vi "harp_read_reg.vi"(0 "port":refnum<visa-resource-name>, 5 "error in (no error)":errorcluster, 6 "port":u8, 8 "reg. address":u8, 9 "type":u8(ring)=1 items=["U8"=1, "U16"=2, "U32 "=4, "U64"=8, "I8"=129, "I16"=130, "I32"=132, "I64"=136, "FLOAT"=68, "BOOL"=17]) -> (10 "HarpDataFrame":T1={"Timestamp(us)"=0.0, "Command"=16, "Error"=FALSE, "Register Address"=16, "Port"=16, "Number of Elements"=16, "Type"=16, "I8"=0, "U8"=0, "U16"=0, "I16"=0, "U32"=0, "I32"=0, "U64"=0, "I64"=0, "Float"=0.0, "U8[]"=[], "I8[]"=[], "U16[]"=[], "I16[]"=[], "U32[]"=[], "I32[]"=[], "U64[]"=[], "I64[]"=[], "Float[]"=[]} {"Timestamp(us)" format="%.6f"}, 11 "timestamp":dbl format="%.6f", 12 "8 bits":u8 format="%x", 13 "bool":bool, 14 "port out":refnum<visa-resource-name>, 15 "16 bits":u16, 16 "32 bits":u32, 17 "64 bits":u64, 18 "float":sgl, 19 "error out":errorcluster)   [LabVIEW 2010]
uses:
  <vilib>/Instr/_visa.llb/VISA Flush IO Buffer Mask.ctl
panel:
  out "Float":sgl
  out "U64":u64
  out "U32":u32
  out "U16":u16
  out "U8":u8
  out "I64":i64
  out "I32":i32
  out "I16":i16
  out "I8":i8
  out "U8[]":u8[](array[numeric])
  out "I8[]":i8[](array[numeric])
  out "U16[]":u16[](array[numeric])
  out "I16[]":i16[](array[numeric])
  out "U32[]":u32[](array[numeric])
  out "I32[]":i32[](array[numeric])
  out "U64[]":u64[](array[numeric])
  out "I64[]":i64[](array[numeric])
  out "Float[]":sgl[](array[numeric])
  in  "Round value":bool
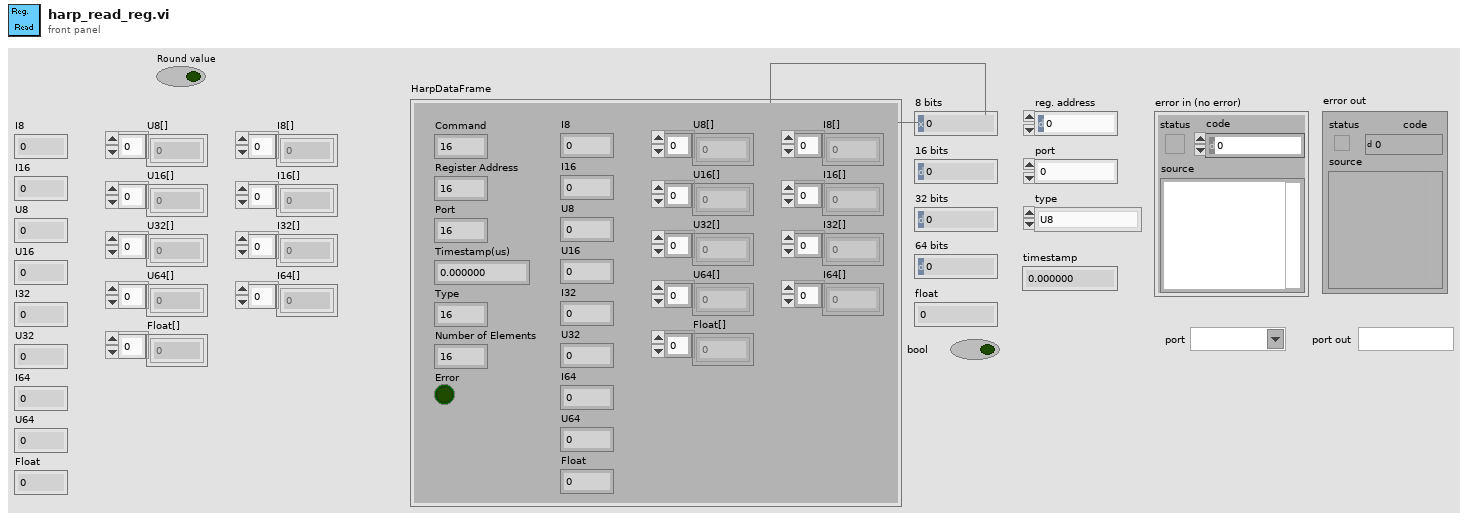
[diagram p1: front panel]
types:
  T1 = cluster{"Timestamp(us)":dbl, "Command":u8, "Error":bool, "Register Address":u8, "Port":u8, "Number of Elements":u8, "Type":u8, "I8":i8, "U8":u8, "U16":u16, "I16":i16, "U32":u32, "I32":i32, "U64":u64, "I64":i64, "Float":sgl, "U8[]":u8[], "I8[]":i8[], "U16[]":u16[], "I16[]":i16[], "U32[]":u32[], "I32[]":i32[], "U64[]":u64[], "I64[]":i64[], "Float[]":sgl[]}
  T2 = typedef "VISA Flush IO Buffer Mask.ctl" = u16
  T3 = enum16{"big-endian, network order", "native, host order", "little-endian"}
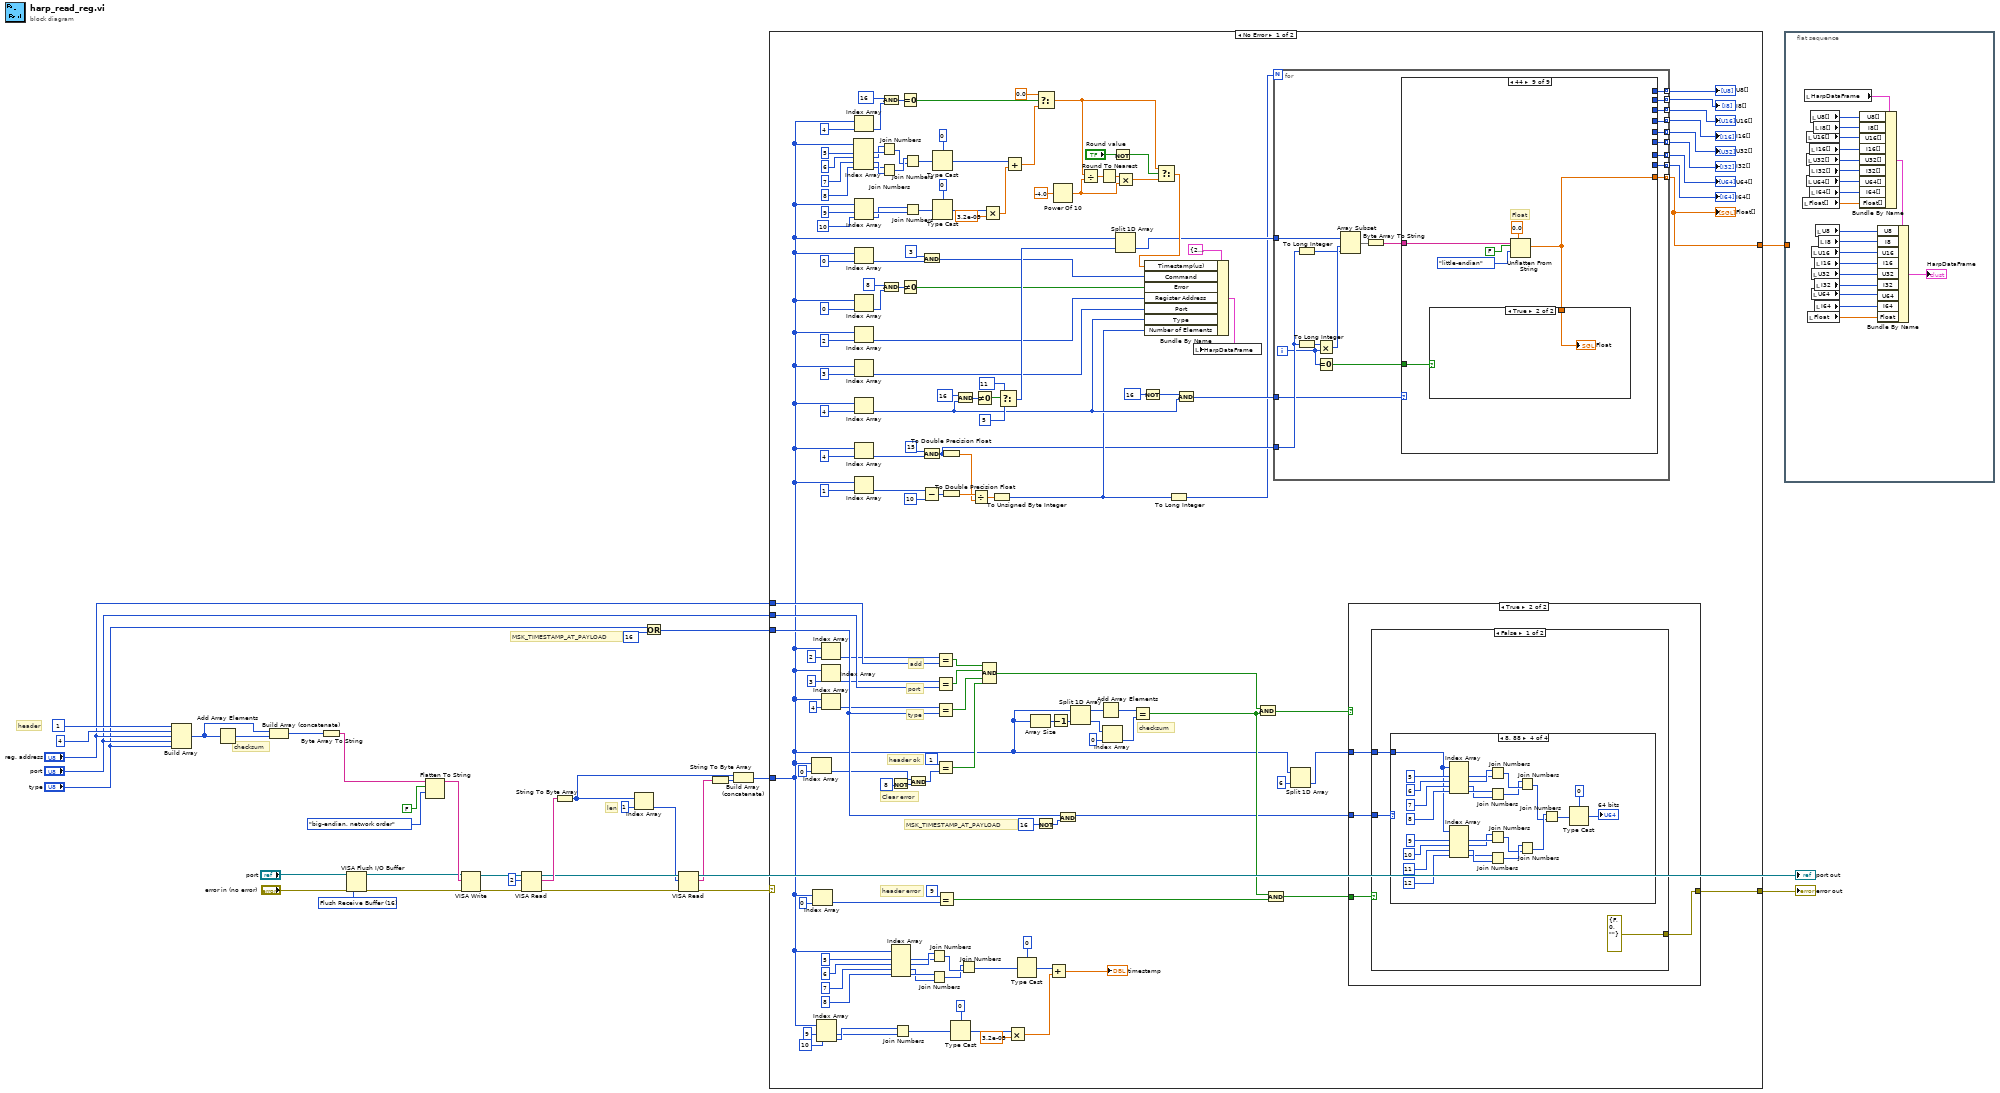
[diagram p0: block diagram]
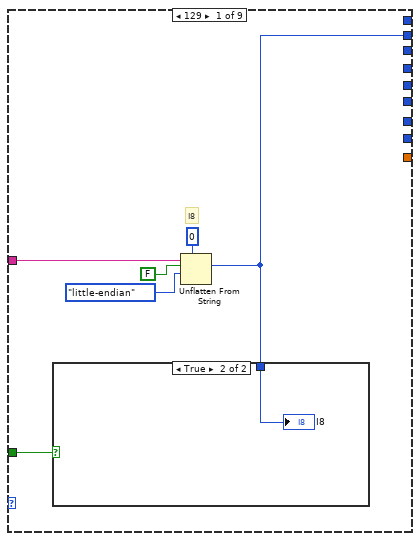
[diagram p2: hidden frame]
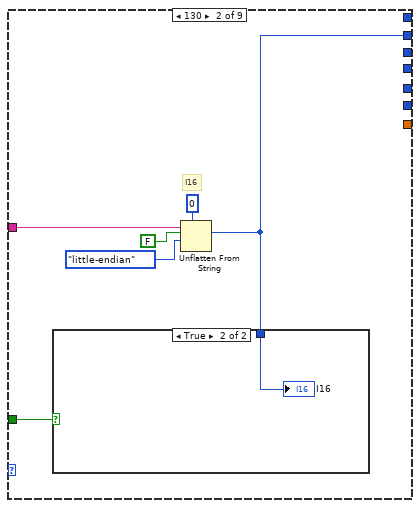
[diagram p4: hidden frame]
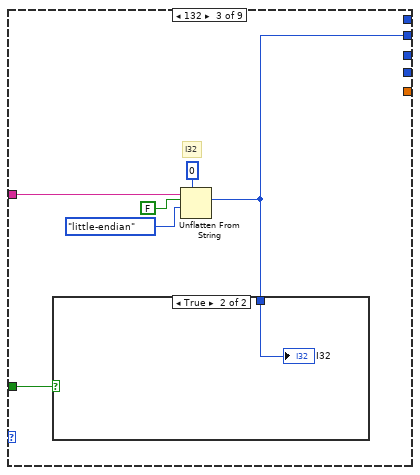
[diagram p6: hidden frame]
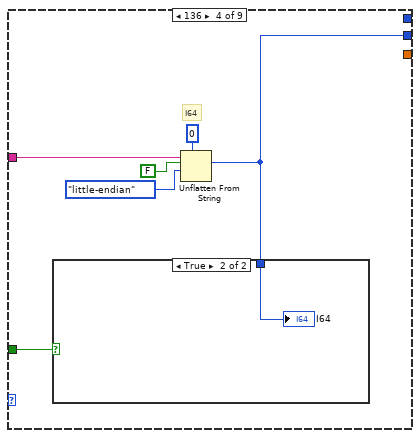
[diagram p8: hidden frame]
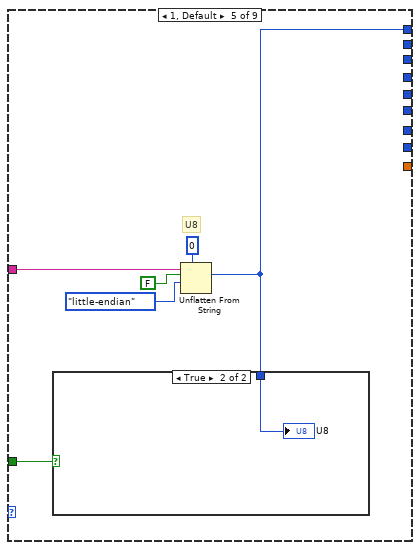
[diagram p10: hidden frame]
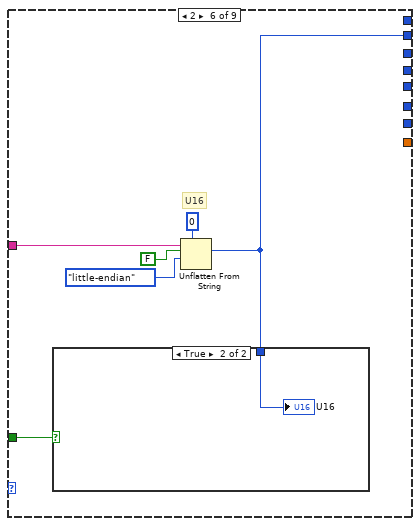
[diagram p12: hidden frame]
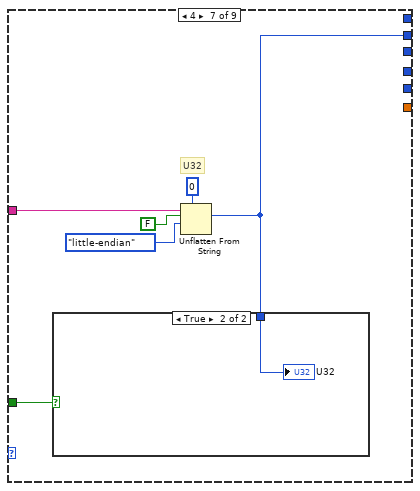
[diagram p14: hidden frame]
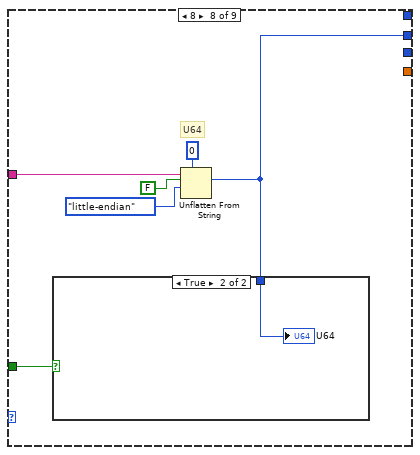
[diagram p16: hidden frame]
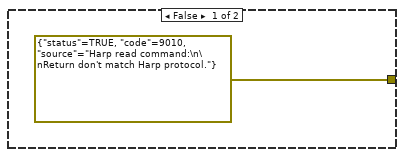
[diagram p19: hidden frame]
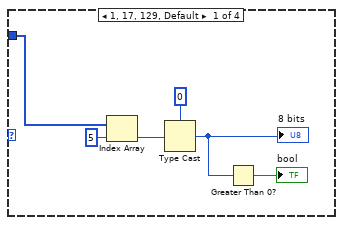
[diagram p20: hidden frame]
diagram:
  w15 = T2 16 items=["Flush Receive Buffer"=16, "Write Transmit Buffer to Device"=32, "Flush Receive Buffer (No I/O)"=64, "Flush Transmit Buffer"=128] ("Mask")
  # "MSK_TIMESTAMP_AT_PAYLOAD"
  # "len"
  # "checksum"
  # "header"
  n1 = Build Array(u8 1 ("element"), u8 4 ("x"), "reg. address", "port", "type") -> (w4:u8[])
  n2 = Add Array Elements(numeric array=w4) -> (sum=w7:u8)
  n3 = Build Array (concatenate)(w4, w7) -> (w6:u8[])
  n4 = Byte Array To String(unsigned byte array=w6) -> (string=w5:string)
  n5 = VISA Flush I/O Buffer(VISA resource name="port", mask (16)=w15, error in (no error)="error in (no error)") -> (VISA resource name out=w12:refnum<visa-resource-name>, error out=w11:errorcluster)
  n6 = Flatten To String(anything=w5, prepend array or string size? (T)=FALSE, byte order (0:big-endian, network order)=T3."big-endian, network order") -> (data string=w33:string)  [unwired: 1 in, 2 out]
  n7 = VISA Write(VISA resource name=w12, write buffer=w33, error in (no error)=w11) -> (VISA resource name out=w31:refnum<visa-resource-name>, error out=w29:errorcluster)  [unwired: 1 out]
  n8 = VISA Read(VISA resource name=w31, byte count=u32 2, error in (no error)=w29) -> (VISA resource name out=w24:refnum<visa-resource-name>, read buffer=w25:string, error out=w23:errorcluster)  [unwired: 1 out]
  n9 = String To Byte Array(string=w25) -> (unsigned byte array=w10:u8[])
  n10 = Index Array(array=w10, index=1) -> (element=w19:u8)
  n11 = Or(x="type", y=u8 16) -> (x .or. y?=w3:u8)
  n12 = VISA Read(VISA resource name=w24, byte count=w19, error in (no error)=w23) -> (VISA resource name out=→"port out":refnum<visa-resource-name>, read buffer=w21:string, error out=w8:errorcluster)  [unwired: 1 out]
  n13 = String To Byte Array(string=w21) -> (unsigned byte array=w20:u8[])
  n14 = Build Array (concatenate)(w10, w20) -> (w9:u8[])
  n15 = case shown="No Error" w8 {
    selector: w8 -> [_ w334]
    tunnel: [w186 w334] -> w28
    tunnel: "reg. address" -> [w183 _]
    tunnel: "port" -> [w182 _]
    tunnel: w3 -> [w181 _]
    tunnel: w9 -> [w37 _]
    tunnel: [w36 _] -> w1
    frame No Error {
      # "Clear error"
      # "MSK_TIMESTAMP_AT_PAYLOAD"
      # "checksum"
      # "type"
      # "port"
      # "add"
      # "header error"
      # "header ok"
      n16 = Index Array(array=w37, index=0) -> (element=w126:u8)
      n17 = Index Array(array=w37, index=0) -> (element=w180:u8)
      n18 = Index Array(array=w37, index #1=9 ("index"), index #2=10 ("index")) -> (element #1=w137:u8, element #2=w138:u8)
      n19 = Index Array(array=w37, index=2) -> (element=w174:u8)
      n20 = Index Array(array=w37, index=3) -> (element=w175:u8)
      n21 = Index Array(array=w37, index=4) -> (element=w176:u8)
      n22 = Index Array(array=w37, index #1=5 ("index"), index #2=6 ("index"), index #3=7 ("index"), index #4=8 ("index")) -> (element #1=w48:u8, element #2=w44:u8, element #3=w47:u8, element #4=w46:u8)
      n23 = Index Array(array=w37, index=4) -> (element=w63:u8)
      n24 = Index Array(array=w37, index #1=9 ("index"), index #2=10 ("index")) -> (element #1=w59:u8, element #2=w58:u8)
      n25 = Index Array(array=w37, index=0) -> (element=w69:u8)
      n26 = Index Array(array=w37, index=0) -> (element=w70:u8)
      n27 = Index Array(array=w37, index=2) -> (element=w99:u8)
      n28 = Index Array(array=w37, index=3) -> (element=w100:u8)
      n29 = Index Array(array=w37, index=4) -> (element=w108:u8)
      n30 = Index Array(array=w37, index=4) -> (element=w77:u8)
      n31 = Index Array(array=w37, index=1) -> (element=w81:u8)
      n32 = Join Numbers(hi=w44, lo=w48) -> ((hi.lo)=w43:u16)
      n33 = Join Numbers(hi=w46, lo=w47) -> ((hi.lo)=w45:u16)
      n34 = And(x=u8 16, y=w63) -> (x .and. y?=w39:u8)
      n35 = And(x=u8 8, y=w70) -> (x .and. y?=w72:u8)
      n36 = Not(x=u8 8 ("y")) -> (.not. x?=w127:u8)
      n37 = Index Array(array=w37, index #1=5 ("index"), index #2=6 ("index"), index #3=7 ("index"), index #4=8 ("index")) -> (element #1=w148:u8, element #2=w152:u8, element #3=w149:u8, element #4=w150:u8)
      n38 = Join Numbers(hi=w138, lo=w137) -> ((hi.lo)=w139:u16)
      n39 = Equal To 0?(x=w39) -> (x = 0?=w64:bool)
      n40 = Not Equal To 0?(x=w72) -> (x != 0?=w98:bool)
      n41 = Join Numbers(hi=w45, lo=w43) -> ((hi.lo)=w53:u32)
      n42 = Join Numbers(hi=w58, lo=w59) -> ((hi.lo)=w57:u16)
      n43 = And(x=w126, y=w127) -> (x .and. y?=w125:u8)
      n44 = And(x=u8 3, y=w69) -> (x .and. y?=w97:u8)
      n45 = And(x=u8 15, y=w77) -> (x .and. y?=w88:u8)
      n46 = Subtract(x=w81, y=u8 10) -> (x-y=w83:u8)
      n47 = Join Numbers(hi=w152, lo=w148) -> ((hi.lo)=w153:u16)
      n48 = Join Numbers(hi=w150, lo=w149) -> ((hi.lo)=w151:u16)
      n49 = Type Cast(type=u32 0 ("byte count"), x=w53) -> (*(type *) &x=w41:u32)
      n50 = Type Cast(type=u16 0 ("byte count"), x=w57) -> (*(type *) &x=w55:u16)
      n51 = Equal?(x=w174, y=w183) -> (x = y?=w169:bool)
      n52 = Equal?(x=w175, y=w182) -> (x = y?=w170:bool)
      n53 = Equal?(x=w176, y=w181) -> (x = y?=w171:bool)
      n54 = Equal?(x=u8 1 ("y"), y=w125) -> (x = y?=w166:bool)
      n55 = Equal?(x=u8 9 ("y"), y=w180) -> (x = y?=w124:bool)
      n56 = To Double Precision Float(number=w88) -> (double precision float=w85:dbl)
      n57 = To Double Precision Float(number=w83) -> (double precision float=w86:dbl)
      n58 = Type Cast(type=u16 0 ("byte count"), x=w139) -> (*(type *) &x=w141:u16)
      n59 = And(x=u8 16, y=w108) -> (x .and. y?=w107:u8)
      n60 = Join Numbers(hi=w151, lo=w153) -> ((hi.lo)=w143:u32)
      n61 = Divide(x=w86, y=w85) -> (x/y=w84:dbl)
      n62 = Not Equal To 0?(x=w107) -> (x != 0?=w109:bool)
      n63 = Compound Arithmetic op=AND(w169, w170, w171, w166) -> (w168:bool)
      n64 = Multiply(x=w55, y=3.2e-05) -> (x*y=w40:dbl)
      n65 = To Unsigned Byte Integer(number=w84) -> (unsigned 8bit integer=w101:u8)
      n66 = Select(t=u8 11, s=w109, f=u8 5) -> (s? t:f=w112:u8)
      n67 = Add(x=w41, y=w40) -> (x+y=w65:dbl)
      n68 = Multiply(x=w141, y=3.2e-05) -> (x*y=w156:dbl)
      n69 = Type Cast(type=u32 0 ("byte count"), x=w143) -> (*(type *) &x=w155:u32)
      n70 = Array Size(array=w37) -> (size(s)=w165:i32)
      n71 = Select(t=0.0, s=w64, f=w65) -> (s? t:f=w120:dbl)
      n72 = Not(x=u8 16 ("y")) -> (.not. x?=w130:u8)
      n73 = Add(x=w155, y=w156) -> (x+y=→"timestamp":dbl)
      n74 = Decrement(x=w165) -> (x-1=w164:i32)
      n75 = Power Of 10(x=-4.0) -> (10^x=w117:dbl)
      n76 = And(x=w181, y=w130) -> (x .and. y?=w131:u8)
      n77 = Split 1D Array(array=w37, index=w164) -> (first subarray=w163:u8[], second subarray=w160:u8[])
      n78 = Divide(x=w120, y=w117) -> (x/y=w115:dbl)
      n79 = Round To Nearest(number=w115) -> (nearest integer value=w116:dbl)
      n80 = Add Array Elements(numeric array=w163) -> (sum=w162:u8)
      n81 = Index Array(array=w160, index=0) -> (element=w159:u8)
      n82 = Not(x="Round value") -> (.not. x?=w123:bool)
      n83 = Multiply(x=w116, y=w117) -> (x*y=w119:dbl)
      n84 = Split 1D Array(array=w37, index=w112) -> (second subarray=w105:u8[])  [unwired: 1 out]
      n85 = Equal?(x=w162, y=w159) -> (x = y?=w157:bool)
      n86 = Not(x=u8 16) -> (.not. x?=w102:u8)
      n87 = Select(t=w120, s=w123, f=w119) -> (s? t:f=w121:dbl)
      n88 = Bundle By Name(cluster=T1 {"Timestamp(us)"=2218.246816, "Command"=1, "Error"=FALSE, "Register Address"=18, "Port"=255, "Number of Elements"=1, "Type"=84, "I8"=0, "U8"=0, "U16"=0, "I16"=0, "U32"=0, "I32"=0, "U64"=0, "I64"=0, "Float"=0.0, "U8[]"=[0], "I8[]"=[0], "U16[]"=[0], "I16[]"=[0], "U32[]"=[0], "I32[]"=[0], "U64[]"=[0], "I64[]"=[0], "Float[]"=[0.0]} ("HarpDataFrame"), "Timestamp(us)"=w121, "Command"=w97, "Error"=w98, "Register Address"=w99, "Port"=w100, "Type"=w108, "Number of Elements"=w101) -> (w113:T1)
      n89 = To Long Integer(number=w101) -> (32bit integer=w87:i32)
      n90 = And(x=w102, y=w108) -> (x .and. y?=w104:u8)
      n91 = local write "HarpDataFrame"(w113) -> ()
      n92 = And(x=w168, y=w157) -> (x .and. y?=w167:bool)
      n93 = And(x=w157, y=w124) -> (x .and. y?=w158:bool)
      n94 = for {
        N: w87 -> [_]
        tunnel: w105 -> [w203]
        tunnel: w88 -> [w202]
        tunnel: w104 -> [w198]
        tunnel: [w195] -> w89 mode=indexing
        tunnel: [w194] -> w90 mode=indexing
        tunnel: [w193] -> w91 mode=indexing
        tunnel: [w192] -> w92 mode=indexing
        tunnel: [w191] -> w93 mode=indexing
        tunnel: [w190] -> w94 mode=indexing
        tunnel: [w189] -> w95 mode=indexing
        tunnel: [w188] -> w96 mode=indexing
        tunnel: [w187] -> w36 mode=indexing
        i -> [w197]
        n95 = To Long Integer(number=w202) -> (32bit integer=w199:i32)
        n96 = To Long Integer(number=w202) -> (32bit integer=w200:i32)
        n97 = Multiply(x=w200, y=w197) -> (x*y=w201:i32)
        n98 = Equal To 0?(x=w197) -> (x = 0?=w196:bool)
        n99 = Array Subset(array=w203, index=w201, length=w199) -> (w204:u8[])
        n100 = Byte Array To String(unsigned byte array=w204) -> (string=w205:string)
        n101 = case shown="44" w198 {
          tunnel: w205 -> [w210 w217 w224 w231 w238 w245 w252 w259 w266]
          tunnel: w196 -> [w207 w214 w221 w228 w235 w242 w249 w256 w263]
          tunnel: [_ _ _ _ w234 _ _ _ _] -> w195
          tunnel: [w206 _ _ _ _ _ _ _ _] -> w194
          tunnel: [_ _ _ _ _ w241 _ _ _] -> w193
          tunnel: [_ w213 _ _ _ _ _ _ _] -> w192
          tunnel: [_ _ _ _ _ _ w248 _ _] -> w191
          tunnel: [_ _ w220 _ _ _ _ _ _] -> w190
          tunnel: [_ _ _ _ _ _ _ w255 _] -> w189
          tunnel: [_ _ _ w227 _ _ _ _ _] -> w188
          tunnel: [_ _ _ _ _ _ _ _ w262] -> w187
          frame 129 {
            # "I8"
            n102 = Unflatten From String(type=i8 0 ("Port"), binary string=w210, data includes array or string size? (T)=FALSE, byte order (0:big-endian, network order)=T3."little-endian") -> (value=w206:i8)  [unwired: 1 in, 2 out]
            n103 = case shown="True" w207 {
              tunnel: w206 -> [_ w212]
              frame False {
              }
              frame True {
                "I8" <- w212
              }
            }
          }
          frame 130 {
            # "I16"
            n104 = Unflatten From String(type=i16 0 ("Port"), binary string=w217, data includes array or string size? (T)=FALSE, byte order (0:big-endian, network order)=T3."little-endian") -> (value=w213:i16)  [unwired: 1 in, 2 out]
            n105 = case shown="True" w214 {
              tunnel: w213 -> [_ w219]
              frame False {
              }
              frame True {
                "I16" <- w219
              }
            }
          }
          frame 132 {
            # "I32"
            n106 = Unflatten From String(type=0 ("Port"), binary string=w224, data includes array or string size? (T)=FALSE, byte order (0:big-endian, network order)=T3."little-endian") -> (value=w220:i32)  [unwired: 1 in, 2 out]
            n107 = case shown="True" w221 {
              tunnel: w220 -> [_ w226]
              frame False {
              }
              frame True {
                "I32" <- w226
              }
            }
          }
          frame 136 {
            # "I64"
            n108 = Unflatten From String(type=i64 0 ("Port"), binary string=w231, data includes array or string size? (T)=FALSE, byte order (0:big-endian, network order)=T3."little-endian") -> (value=w227:i64)  [unwired: 1 in, 2 out]
            n109 = case shown="True" w228 {
              tunnel: w227 -> [_ w233]
              frame False {
              }
              frame True {
                "I64" <- w233
              }
            }
          }
          frame 1, Default {
            # "U8"
            n110 = Unflatten From String(type=u8 0 ("Port"), binary string=w238, data includes array or string size? (T)=FALSE, byte order (0:big-endian, network order)=T3."little-endian") -> (value=w234:u8)  [unwired: 1 in, 2 out]
            n111 = case shown="True" w235 {
              tunnel: w234 -> [_ w240]
              frame False {
              }
              frame True {
                "U8" <- w240
              }
            }
          }
          frame 2 {
            # "U16"
            n112 = Unflatten From String(type=u16 0 ("Port"), binary string=w245, data includes array or string size? (T)=FALSE, byte order (0:big-endian, network order)=T3."little-endian") -> (value=w241:u16)  [unwired: 1 in, 2 out]
            n113 = case shown="True" w242 {
              tunnel: w241 -> [_ w247]
              frame False {
              }
              frame True {
                "U16" <- w247
              }
            }
          }
          frame 4 {
            # "U32"
            n114 = Unflatten From String(type=u32 0 ("Port"), binary string=w252, data includes array or string size? (T)=FALSE, byte order (0:big-endian, network order)=T3."little-endian") -> (value=w248:u32)  [unwired: 1 in, 2 out]
            n115 = case shown="True" w249 {
              tunnel: w248 -> [_ w254]
              frame False {
              }
              frame True {
                "U32" <- w254
              }
            }
          }
          frame 8 {
            # "U64"
            n116 = Unflatten From String(type=u64 0 ("Port"), binary string=w259, data includes array or string size? (T)=FALSE, byte order (0:big-endian, network order)=T3."little-endian") -> (value=w255:u64)  [unwired: 1 in, 2 out]
            n117 = case shown="True" w256 {
              tunnel: w255 -> [_ w261]
              frame False {
              }
              frame True {
                "U64" <- w261
              }
            }
          }
          frame 68 {
            # "Float"
            n118 = Unflatten From String(type=sgl 0.0 ("Port"), binary string=w266, data includes array or string size? (T)=FALSE, byte order (0:big-endian, network order)=T3."little-endian") -> (value=w262:sgl)  [unwired: 1 in, 2 out]
            n119 = case shown="True" w263 {
              tunnel: w262 -> [_ w268]
              frame False {
              }
              frame True {
                "Float" <- w268
              }
            }
          }
        }
      }
      "U8[]" <- w89
      "I8[]" <- w90
      "U16[]" <- w91
      "I16[]" <- w92
      "U32[]" <- w93
      "I32[]" <- w94
      "U64[]" <- w95
      "I64[]" <- w96
      "Float[]" <- w36
      n120 = Split 1D Array(array=w37, index=6) -> (second subarray=w132:u8[])  [unwired: 1 out]
      n121 = case shown="True" w167 {
        tunnel: [errorcluster {"status"=TRUE, "code"=9010, "source"="Harp read command:\n\nReturn don't match Harp protocol."} ("error out") w270] -> w186
        tunnel: w131 -> [_ w273]
        tunnel: w132 -> [_ w272]
        tunnel: w158 -> [_ w271]
        frame False {
        }
        frame True {
          n122 = case shown="False" w271 {
            tunnel: w273 -> [w276 _]
            tunnel: w272 -> [w275 _]
            tunnel: [errorcluster {"status"=FALSE, "code"=0, "source"=""} ("error out") errorcluster {"status"=TRUE, "code"=9010, "source"="Harp read command:\n\nDevice report an error when reading."} ("error out")] -> w270
            frame False {
              n123 = case shown="8, 88" w276 {
                tunnel: w275 -> [w280 w285 w295 w312]
                frame 1, 17, 129, Default {
                  n124 = Index Array(array=w280, index=5) -> (element=w281:u8)
                  n125 = Type Cast(type=u8 0 ("byte count"), x=w281) -> (*(type *) &x=w277:u8)
                  "8 bits" <- w277
                  n126 = Greater Than 0?(x=w277) -> (x > 0?=→"bool":bool)
                }
                frame 2, 130 {
                  n127 = Index Array(array=w285, index #1=5 ("index"), index #2=6 ("index")) -> (element #1=w286:u8, element #2=w287:u8)
                  n128 = Join Numbers(hi=w287, lo=w286) -> ((hi.lo)=w289:u16)
                  n129 = Type Cast(type=u16 0 ("byte count"), x=w289) -> (*(type *) &x=→"16 bits":u16)
                }
                frame 4, 68, 132 {
                  n130 = Index Array(array=w295, index #1=5 ("index"), index #2=6 ("index"), index #3=7 ("index"), index #4=8 ("index")) -> (element #1=w300:u8, element #2=w304:u8, element #3=w301:u8, element #4=w302:u8)
                  n131 = Join Numbers(hi=w304, lo=w300) -> ((hi.lo)=w305:u16)
                  n132 = Join Numbers(hi=w302, lo=w301) -> ((hi.lo)=w303:u16)
                  n133 = Join Numbers(hi=w303, lo=w305) -> ((hi.lo)=w292:u32)
                  n134 = Type Cast(type=sgl 0.0 ("byte count"), x=w292) -> (*(type *) &x=→"float":sgl)
                  n135 = Type Cast(type=u32 0 ("byte count"), x=w292) -> (*(type *) &x=→"32 bits":u32)
                }
                frame 8, 136 {
                  n136 = Index Array(array=w312, index #1=5 ("index"), index #2=6 ("index"), index #3=7 ("index"), index #4=8 ("index")) -> (element #1=w327:u8, element #2=w331:u8, element #3=w328:u8, element #4=w329:u8)
                  n137 = Index Array(array=w312, index #1=9 ("index"), index #2=10 ("index"), index #3=11 ("index"), index #4=12 ("index")) -> (element #1=w318:u8, element #2=w314:u8, element #3=w317:u8, element #4=w316:u8)
                  n138 = Join Numbers(hi=w331, lo=w327) -> ((hi.lo)=w332:u16)
                  n139 = Join Numbers(hi=w329, lo=w328) -> ((hi.lo)=w330:u16)
                  n140 = Join Numbers(hi=w314, lo=w318) -> ((hi.lo)=w313:u16)
                  n141 = Join Numbers(hi=w316, lo=w317) -> ((hi.lo)=w315:u16)
                  n142 = Join Numbers(hi=w330, lo=w332) -> ((hi.lo)=w310:u32)
                  n143 = Join Numbers(hi=w315, lo=w313) -> ((hi.lo)=w311:u32)
                  n144 = Join Numbers(hi=w311, lo=w310) -> ((hi.lo)=w308:u64)
                  n145 = Type Cast(type=u64 0 ("byte count"), x=w308) -> (*(type *) &x=→"64 bits":u64)
                }
              }
            }
            frame True {
            }
          }
        }
      }
    }
    frame Error {
    }
  }
  "error out" <- w28
  n146 = flat-sequence {
    tunnel: w1 -> [_]
    frame #0 {
      n147 = local read "Float[]"() -> (w347:sgl[])
      n148 = local read "HarpDataFrame"() -> (w336:T1)
      n149 = local read "U16[]"() -> (w353:u16[])
      n150 = local read "U32[]"() -> (w351:u32[])
      n151 = local read "U64[]"() -> (w349:u64[])
      n152 = local read "Float"() -> (w337:sgl)
      n153 = local read "I16[]"() -> (w352:i16[])
      n154 = local read "I32[]"() -> (w350:i32[])
      n155 = local read "I64[]"() -> (w348:i64[])
      n156 = local read "U8[]"() -> (w355:u8[])
      n157 = local read "U16"() -> (w343:u16)
      n158 = local read "U32"() -> (w341:u32)
      n159 = local read "U64"() -> (w339:u64)
      n160 = local read "I8[]"() -> (w354:i8[])
      n161 = local read "I16"() -> (w342:i16)
      n162 = local read "I32"() -> (w340:i32)
      n163 = local read "I64"() -> (w338:i64)
      n164 = local read "U8"() -> (w345:u8)
      n165 = local read "I8"() -> (w344:i8)
      n166 = Bundle By Name(cluster=w336, "U8[]"=w355, "I8[]"=w354, "U16[]"=w353, "I16[]"=w352, "U32[]"=w351, "I32[]"=w350, "U64[]"=w349, "I64[]"=w348, "Float[]"=w347) -> (w346:T1)
      n167 = Bundle By Name(cluster=w346, "U8"=w345, "I8"=w344, "U16"=w343, "I16"=w342, "U32"=w341, "I32"=w340, "U64"=w339, "I64"=w338, "Float"=w337) -> (→"HarpDataFrame":T1)
    }
  }
